vi "Data Get Pk2Pk.vi"(11 "Data":dbl[](array[numeric])) -> (4 "XY Graph":cluster{"X":dbl[], "Y":dbl[]}[](graph))   [LabVIEW 2020]
panel:
  out "max value":dbl
  out "Waveform Graph 4":waveform(dbl)(graph)
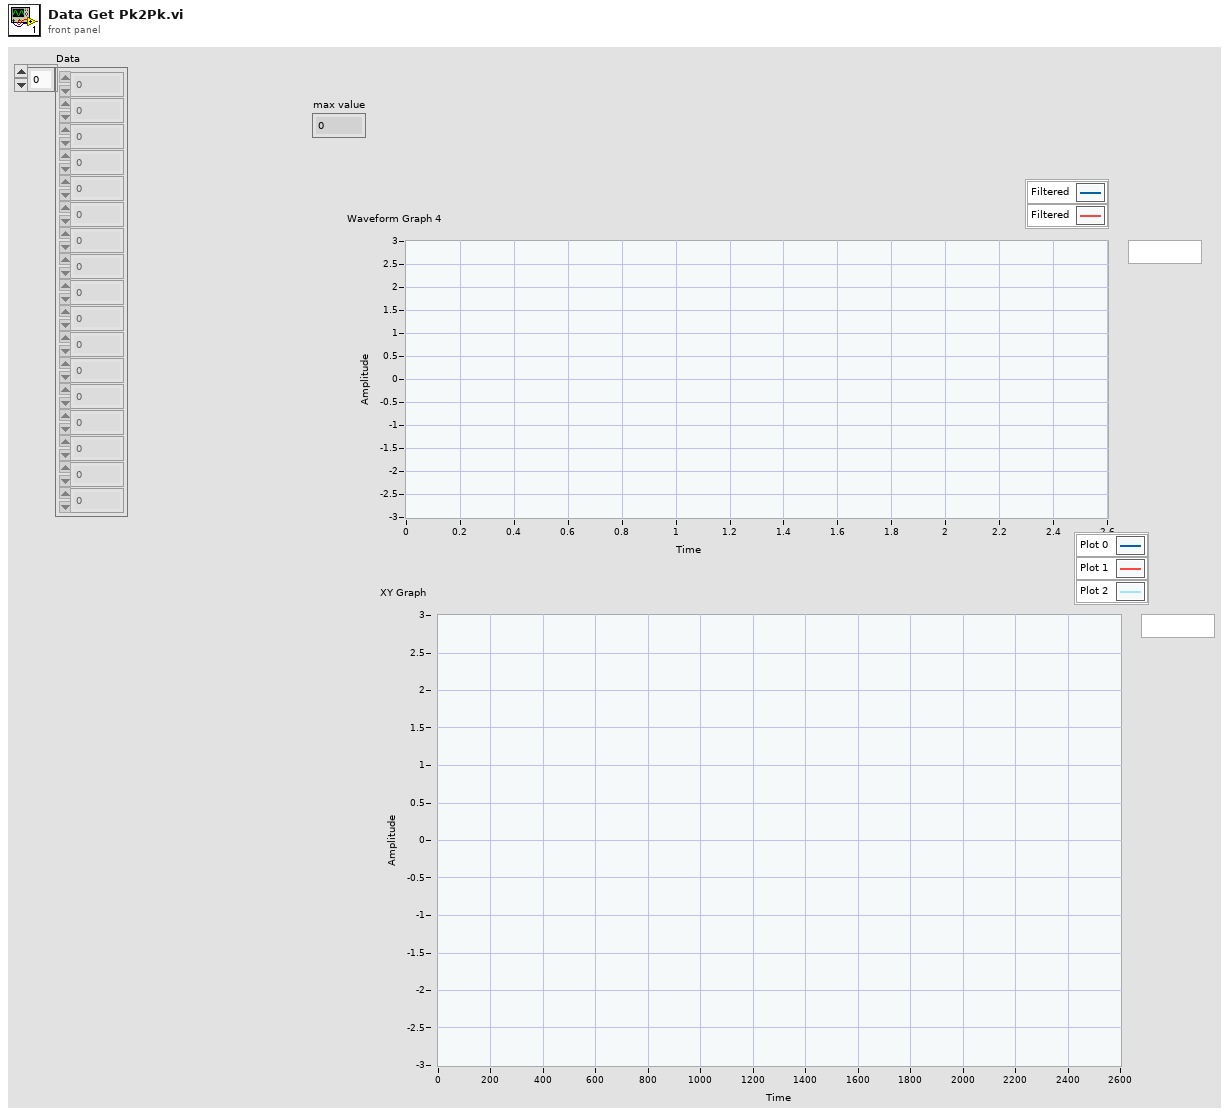
[diagram p1: front panel]
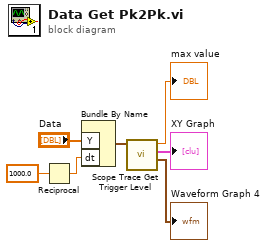
[diagram p0: block diagram]
diagram:
  n1 = Reciprocal(x=1000.0 ("mean")) -> (1/x=w6:dbl)
  n2 = Bundle By Name("Y"="Data", "dt"=w6) -> (w4:waveform(dbl))  [unwired: 1 in]
  n3 = call "Scope Trace Get Trigger Level.vi"("Waveform Data"=w4) -> ("Waveform Graph 2"=→"Waveform Graph 4":waveform(dbl), "XY Graph"=→"XY Graph":cluster{"X":dbl[], "Y":dbl[]}[], "max value"=→"max value":dbl)  [unwired: 8 in]
